vi "Send Command.vi"(8 "error in (no error)":errorcluster, 10 "Command":string, 11 "addr":refnum<visa-resource-name>) -> (0 "error out":errorcluster, 3 "addr dup":refnum<visa-resource-name>)   [LabVIEW 2024, in "FW Arduino Control.lvclass"]
uses:
  FW Arduino Control.lvclass
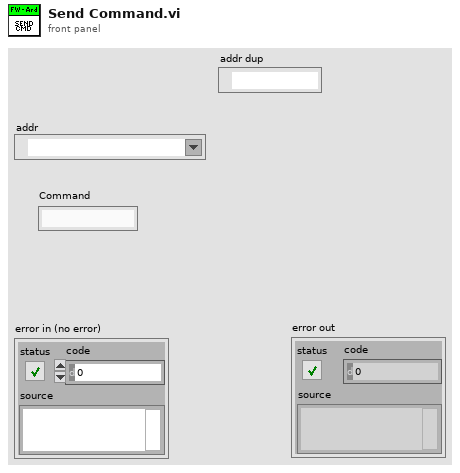
[diagram p1: front panel]
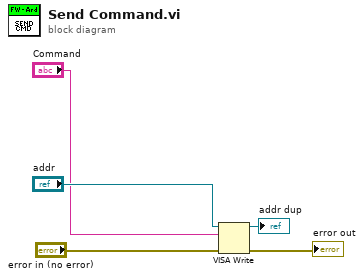
[diagram p0: block diagram]
diagram:
  n1 = VISA Write(VISA resource name="addr", write buffer="Command", error in (no error)="error in (no error)") -> (VISA resource name out=→"addr dup":refnum<visa-resource-name>, error out=→"error out":errorcluster)  [unwired: 1 out]
